vi "DISPENSADOR DE BEBIDAS.vi"() -> ()   [LabVIEW 2020]
uses:
  <vilib>/userdefined/High Color/IMAQdx.ctl
  <vilib>/MakerHub/LINX/Public/Peripherals/Digital/Digital Write N Chans.vi
  <vilib>/MakerHub/LINX/Public/Peripherals/Digital/Digital Write 1 Chan.vi
  <vilib>/MakerHub/LINX/Private/Local IO/LinxDigitalWrite.vi
  <vilib>/MakerHub/LINX/Public/Utilities/Check Channel.vi
  <vilib>/MakerHub/LINX/Public/Utilities/Open Serial.vi
  <vilib>/MakerHub/LINX/Private/Utilties/Generate Error.vi
  <vilib>/vision/driver/NI_Vision_Acquisition_Software.lvlib
  <vilib>/vision/NI_Vision_Development_Module.lvlib
  <vilib>/MakerHub/LINX/LMH-LINX.lvlib
panel:
  in  "path 3":path
  in  "path 2":path
  in  "path":path
  in  "stop":bool
  out "SPRITE":bool
  out "Image 2":T1(plugin-control)
  out "FANTA":bool
  out "COCA-COLA":bool
  in  "Session In":T2
  in  "TAMAÑO":dbl=3.0 caption="Delay Time (s)"
  out "SABOR":string
  out "FRECUENCIA":u32
  in  "SERIAL PORT":refnum<visa-resource-name>="N/A"
  out "tres":bool
  out "dos":bool
  out "uno":bool
  out "Found?":bool
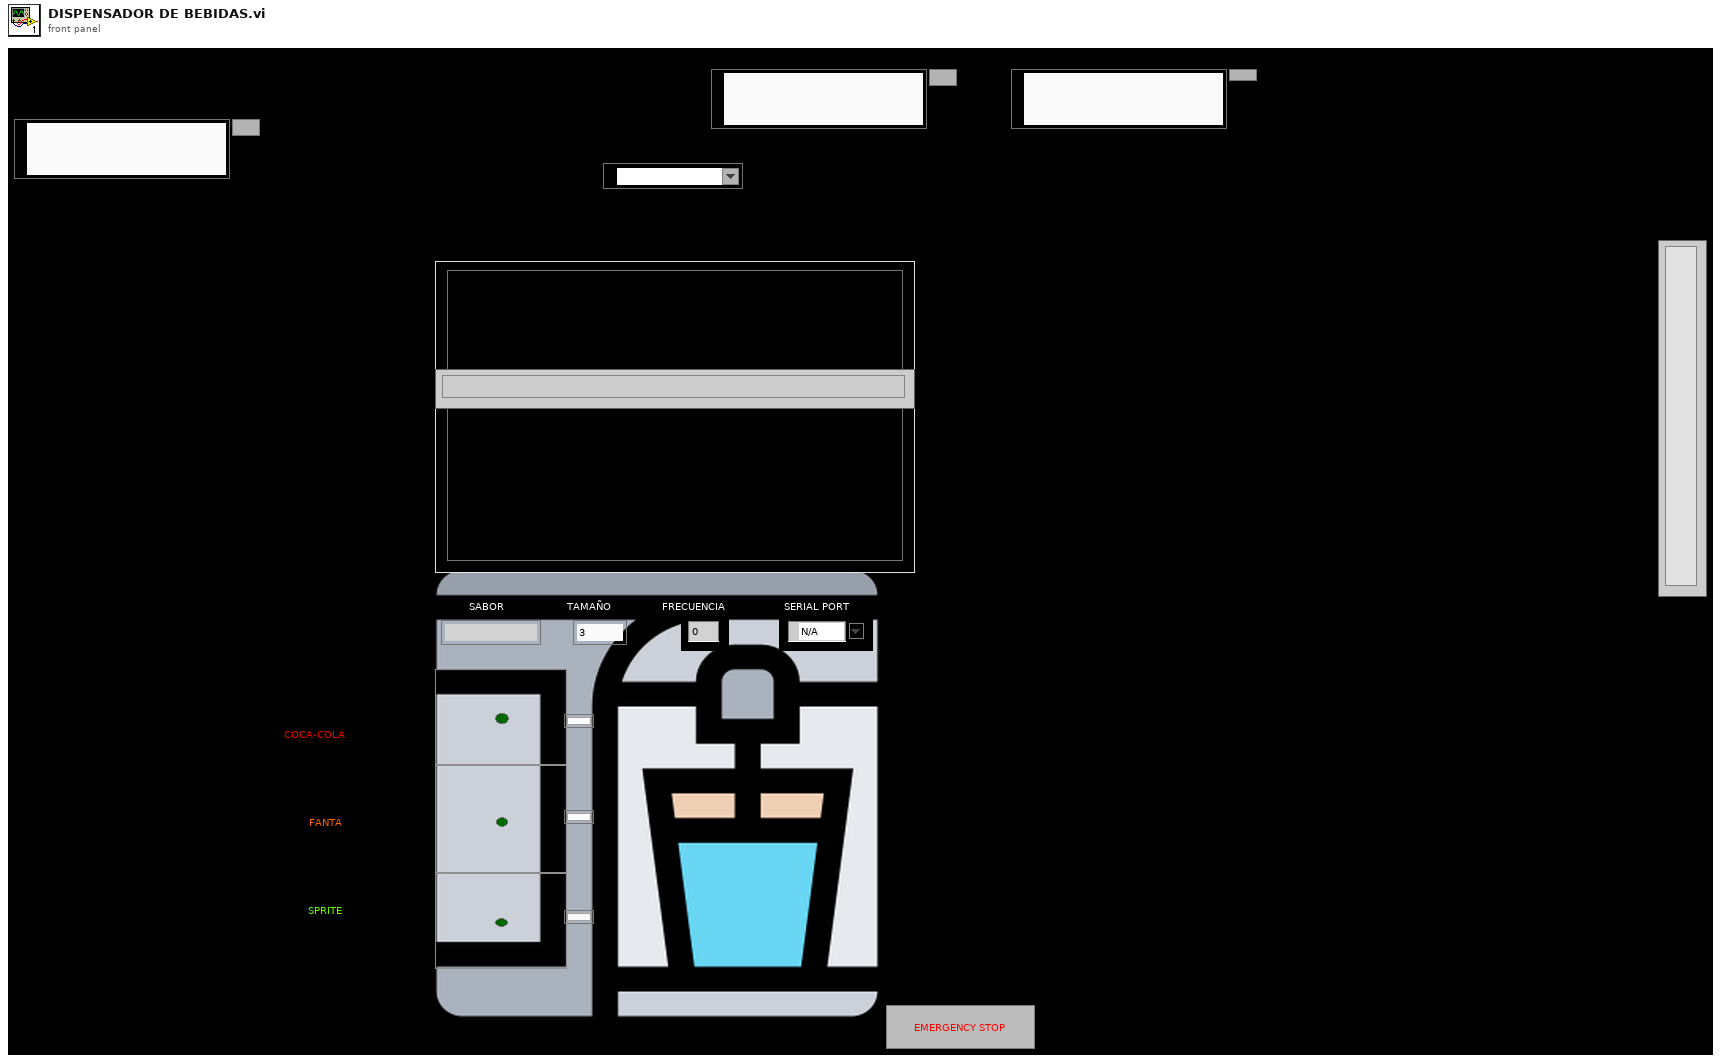
[diagram p1: front panel]
types:
  T1 = typedef "IMAQ Image.ctl" = refnum<image>
  T2 = typedef "IMAQdx.ctl" = refnum<k21>
  T3 = typedef "LMH-LINX.lvlib/LINX Ref.ctl" = cluster{"IO":T4, "Interface":T5, "LINX Device Config":T6}
  T4 = typedef "LMH-LINX.lvlib/Platform.ctl" = enum16{"Remote", "Local"}
  T5 = typedef "LMH-LINX.lvlib/Interface.ctl" = enum16{"Serial", "TCP"}
  T6 = typedef "LMH-LINX.lvlib/Device.lvlib/LINX Device Config.ctl" = cluster{"Interface":T5, "COM Port":refnum<visa-resource-name>, "TCP Configuration":T7, "Device Family":u8, "Device ID":u8, "Device Name":string, "TCP Ref":refnum<k5>, "Channels":T8}
  T7 = typedef "LMH-LINX.lvlib/Device.lvlib/TCP Config.ctl" = cluster{"IP Address":string, "Port":u16}
  T8 = typedef "LMH-LINX.lvlib/Channels.ctl" = cluster{"DI":u8[], "DO":u8[], "AI":u8[], "AO":u8[], "PWM":u8[], "QE":u8[], "UART":u8[], "I2C 2":u8[], "SPI":u8[], "CAN":u8[], "Servo":u8[], "AI Ref (V)":dbl, "AI Resolution (Bits)":u8, "AO Ref (V)":dbl, "AO Resolution (Bits)":u8}
  T9 = typedef "QR Code Report.ctl" = cluster{"Found?":bool, "Data":string, "Bounding Box":cluster{"x":sgl, "y":sgl}[], "Errors Corrected":u32, "Dimensions (Rows/Cols)":u32, "Version":u32, "QR Model":T10, "Stream Mode":T11, "Barcode Polarity":T12, "Mirrored?":bool, "Append Stream Position":u32, "Size of Append Stream":u32, "First EAN-128 ID":i32, "First Alternate Language ID":i32, "Append Stream ID":u32, "Minimum Edge Strength":u32, "Demodulation Mode":T13, "Cell Sample Size":T14, "Cell Filter Mode":T15}
  T10 = typedef "QR Code Model Type.ctl" = i32
  T11 = typedef "QR Code Stream Mode Type.ctl" = i32
  T12 = typedef "Data Matrix Polarity.ctl" = i32
  T13 = typedef "Demodulation Mode.ctl" = i32
  T14 = typedef "Cell Sample Size.ctl" = i32
  T15 = typedef "Cell Filter Mode.ctl" = i32
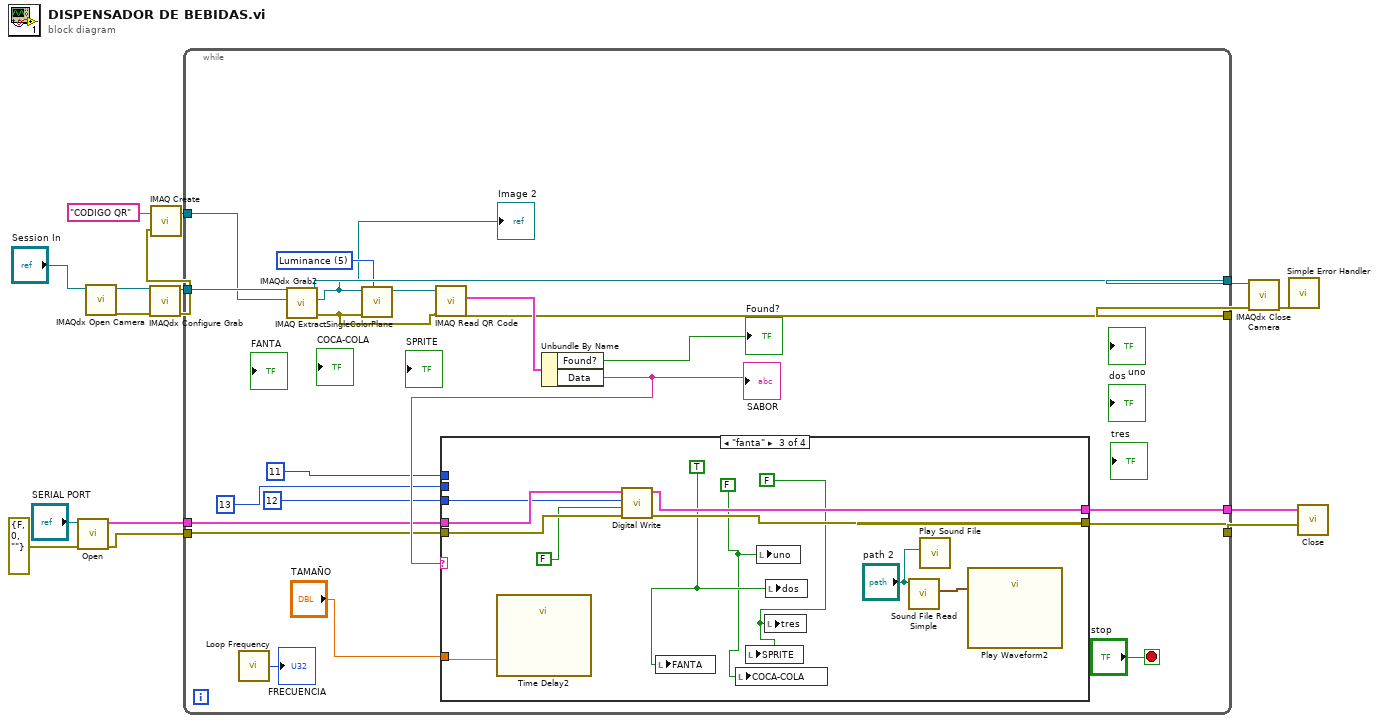
[diagram p0: block diagram]
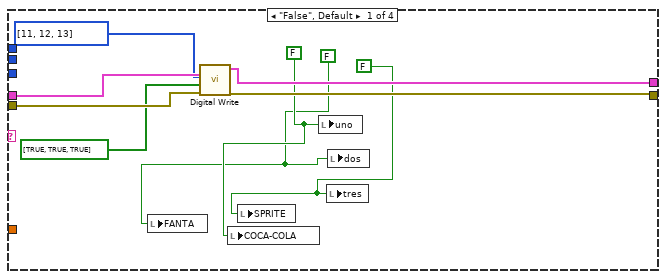
[diagram p2: hidden frame]
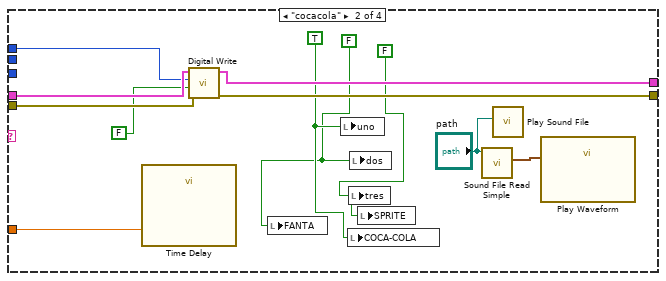
[diagram p3: hidden frame]
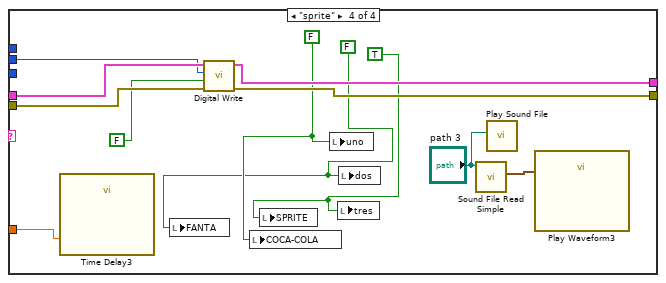
[diagram p4: hidden frame]
diagram:
  n1 = call-poly <vilib>:"Open.vi"("Error In"=errorcluster {"status"=FALSE, "code"=0, "source"=""}, "Serial Port"="SERIAL PORT") -> ("Error Out"=w3:errorcluster, "LINX Resource"=w4:T3)  [unwired: 7 in, 1 out]
  n2 = call <vilib>:"IMAQdx Open Camera.vi"("Session In"="Session In") -> ("error out"=w15:errorcluster, "Session Out"=w16:T2)  [unwired: 9 in]
  n3 = call <vilib>:"IMAQdx Configure Grab.vi"("error in"=w15, "Session In"=w16) -> ("error out"=w13:errorcluster, "Session Out"=w11:T2)  [unwired: 8 in]
  n4 = call "IMAQ Create"("Image Name"="CODIGO QR", "error in (no error)"=w13) -> ("New Image"=w10:T1)  [unwired: 3 in, 1 out]
  n5 = while {
    tunnel: w11 -> [w37]
    tunnel: w10 -> [w36]
    tunnel: [w32] -> w9
    tunnel: [w31] -> w8
    tunnel: w4 -> [w26]
    tunnel: w3 -> [w25]
    tunnel: [w24] -> w2
    tunnel: [w23] -> w1
    stop <- "stop" stop-if-true
    w30 = 5 items=["Red", "Green", "Blue", "Hue", "Saturation", "Luminance", "Value", "Intensity"] ("Color Plane")
    n6 = call <vilib>:"Loop Frequency.vi"() -> ("Loop Rate (Hz)"=→"FRECUENCIA":u32)
    n7 = call <vilib>:"IMAQdx Grab2.vi"("Image In"=w36, "Session In"=w37) -> ("error out"=w34:errorcluster, "Image Out"=w18:T1, "Session Out"=w32:T2)  [unwired: 6 in, 1 out]
    "Image 2" <- w18
    n8 = call "IMAQ ExtractSingleColorPlane"("Color Plane"=w30, "error in (no error)"=w34, "Image Src"=w18) -> ("Image Dst Out"=w35:T1)  [unwired: 7 in, 1 out]
    n9 = call "IMAQ Read QR Code"("error in (no error)"=w34, "Image"=w35) -> ("error out"=w31:errorcluster, "QR Code Report"=w33:T9)  [unwired: 6 in, 2 out]
    n10 = Unbundle By Name(w33) -> ("Found?"=→"Found?":bool, "Data"=w27:string)
    "SABOR" <- w27
    n11 = case shown="\"fanta\"" w27 {
      tunnel: w26 -> [w46 w58 w70 w81]
      tunnel: w25 -> [w45 w57 w69 w80]
      tunnel: [w44 w56 w68 w78] -> w24
      tunnel: [w43 w55 w67 w77] -> w23
      tunnel: 11 -> [_ w54 _ _]
      tunnel: 12 -> [_ _ w66 _]
      tunnel: "TAMAÑO" -> [_ w53 w65 w82]
      tunnel: 13 -> [_ _ _ w79]
      frame "False", Default {
        w38 = FALSE
        w39 = FALSE
        w40 = FALSE
        n12 = local write "FANTA"(w39) -> ()
        n13 = call-poly <vilib>:"Digital Write.vi"("Error In"=w45, "Values"=bool[] [TRUE, TRUE, TRUE], "DO Channels"=i32[] [11, 12, 13], "LINX Resource"=w46) -> ("Error Out"=w43:errorcluster, "LINX Resource"=w44:T3)  [unwired: 6 in]
        n14 = local write "COCA-COLA"(w40) -> ()
        n15 = local write "SPRITE"(w38) -> ()
        n16 = local write "uno"(w40) -> ()
        n17 = local write "tres"(w38) -> ()
        n18 = local write "dos"(w39) -> ()
      }
      frame "cocacola" {
        w50 = FALSE
        w49 = FALSE
        w51 = TRUE
        n19 = call "Time Delay"("Delay Time (s)"=w53) -> ()  [unwired: 10 in, 1 out]
        n20 = call-poly <vilib>:"Digital Write.vi"("Error In"=w57, "Output Value"=FALSE, "DO Channel"=w54, "LINX Resource"=w58) -> ("Error Out"=w55:errorcluster, "LINX Resource"=w56:T3)  [unwired: 6 in]
        n21 = local write "FANTA"(w49) -> ()
        n22 = local write "uno"(w51) -> ()
        n23 = local write "COCA-COLA"(w51) -> ()
        n24 = local write "tres"(w50) -> ()
        n25 = local write "dos"(w49) -> ()
        n26 = local write "SPRITE"(w50) -> ()
        n27 = call <vilib>:"Sound File Read Simple.vi"("path"="path") -> ("data"=w48:waveform(dbl)[])  [unwired: 7 in, 3 out]
        n28 = call <vilib>:"Play Sound File.vi"("path"="path") -> ()  [unwired: 9 in, 2 out]
        n29 = call "Play Waveform"("Data"=w48) -> ()  [unwired: 18 in, 1 out]
      }
      frame "fanta" {
        w61 = FALSE
        w62 = FALSE
        w63 = TRUE
        n30 = call "Time Delay2"("Delay Time (s)"=w65) -> ()  [unwired: 10 in, 1 out]
        n31 = call-poly <vilib>:"Digital Write.vi"("Error In"=w69, "Output Value"=FALSE, "DO Channel"=w66, "LINX Resource"=w70) -> ("Error Out"=w67:errorcluster, "LINX Resource"=w68:T3)  [unwired: 6 in]
        n32 = local write "FANTA"(w63) -> ()
        n33 = local write "COCA-COLA"(w62) -> ()
        n34 = local write "SPRITE"(w61) -> ()
        n35 = local write "uno"(w62) -> ()
        n36 = local write "tres"(w61) -> ()
        n37 = local write "dos"(w63) -> ()
        n38 = call <vilib>:"Sound File Read Simple.vi"("path"="path 2") -> ("data"=w60:waveform(dbl)[])  [unwired: 7 in, 3 out]
        n39 = call <vilib>:"Play Sound File.vi"("path"="path 2") -> ()  [unwired: 9 in, 2 out]
        n40 = call "Play Waveform2"("Data"=w60) -> ()  [unwired: 18 in, 1 out]
      }
      frame "sprite" {
        w73 = FALSE
        w74 = FALSE
        w75 = TRUE
        n41 = call "Time Delay3"("Delay Time (s)"=w82) -> ()  [unwired: 10 in, 1 out]
        n42 = local write "FANTA"(w73) -> ()
        n43 = call-poly <vilib>:"Digital Write.vi"("Error In"=w80, "Output Value"=FALSE, "DO Channel"=w79, "LINX Resource"=w81) -> ("Error Out"=w77:errorcluster, "LINX Resource"=w78:T3)  [unwired: 6 in]
        n44 = local write "COCA-COLA"(w74) -> ()
        n45 = local write "SPRITE"(w75) -> ()
        n46 = local write "uno"(w74) -> ()
        n47 = local write "tres"(w75) -> ()
        n48 = local write "dos"(w73) -> ()
        n49 = call <vilib>:"Sound File Read Simple.vi"("path"="path 3") -> ("data"=w72:waveform(dbl)[])  [unwired: 7 in, 3 out]
        n50 = call <vilib>:"Play Sound File.vi"("path"="path 3") -> ()  [unwired: 9 in, 2 out]
        n51 = call "Play Waveform3"("Data"=w72) -> ()  [unwired: 18 in, 1 out]
      }
    }
  }
  n52 = call <vilib>:"IMAQdx Close Camera.vi"("error in"=w8, "Session In"=w9) -> ("error out"=w7:errorcluster)  [unwired: 9 in]
  n53 = call <vilib>:"Simple Error Handler.vi"("error in (no error)"=w7) -> ()  [unwired: 4 in, 5 out]
  n54 = call <vilib>:"Close.vi"("Error In"=w1, "LINX Resource"=w2) -> ()  [unwired: 9 in, 1 out]
